vi "ImageGrabStatus.vi"(8 "error in (no error)":errorcluster, 11 "Image in":refnum<class "Image.lvclass">) -> (0 "error out":errorcluster, 2 "Stop?":bool, 3 "Image out":refnum<class "Image.lvclass">)   [LabVIEW 2012, in "Image.lvclass"]
uses:
  classes/Image.lvclass
  classes/Image.lvclass/Image.ctl
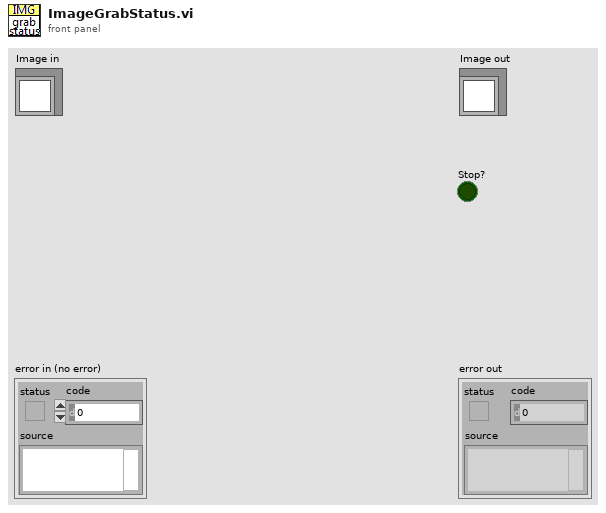
[diagram p1: front panel]
types:
  T1 = typedef "ScanMode.ctl" = enum16{"None", "Continuous", "Point Scan (CH3 cursor)", "Point Scan Move (CH3 cursor)", "Grab", "Grab Move Stage", "Grab Move Z-stage", "Cont. Move Z-stage", "Spec Move Stage", "Spec Move Cont", "Surf Calib"}
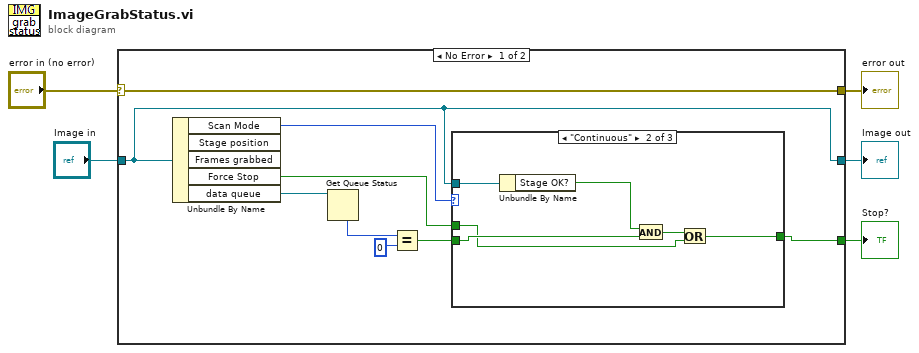
[diagram p0: block diagram]
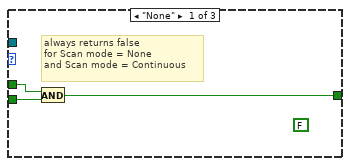
[diagram p2: hidden frame]
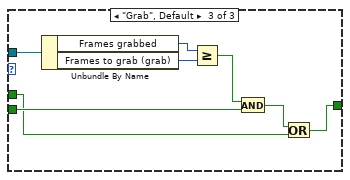
[diagram p3: hidden frame]
diagram:
  n1 = case shown="No Error" "error in (no error)" {
    selector: "error in (no error)" -> [w14 w33]
    tunnel: [w14 w33] -> w4
    tunnel: [w13 w32] -> w2
    tunnel: "Image in" -> [w13 w32]
    tunnel: [w6 _] -> w1
    frame No Error {
      n2 = Unbundle By Name(w13) -> ("Scan Mode"=w12:T1, "Force Stop"=w11:bool, "data queue"=w10:refnum<queue>)  [unwired: 2 out]
      n3 = Get Queue Status(queue=w10) -> (# elements in queue=w9:i32)  [unwired: 2 in, 7 out]
      n4 = Equal?(x=w9, y=0) -> (x = y?=w7:bool)
      n5 = case shown="\"Continuous\"" w12 {
        tunnel: [w15 w18 w24] -> w6
        tunnel: w13 -> [_ w23 w29]
        tunnel: w11 -> [w17 w19 w25]
        tunnel: w7 -> [w16 w21 w27]
        frame "None" {
          (unwired) FALSE
          # "always returns false\nfor Scan mode = None\nand Scan mode = Continuous"
          n6 = And(x=w17, y=w16) -> (x .and. y?=w15:bool)
        }
        frame "Continuous" {
          n7 = Unbundle By Name(w23) -> ("Stage OK?"=w22:bool)
          n8 = And(x=w22, y=w21) -> (x .and. y?=w20:bool)
          n9 = Or(x=w20, y=w19) -> (x .or. y?=w18:bool)
        }
        frame "Grab", Default {
          n10 = Unbundle By Name(w29) -> ("Frames grabbed"=w31:i32, "Frames to grab (grab)"=w30:i32)
          n11 = Greater Or Equal?(x=w31, y=w30) -> (x >= y?=w28:bool)
          n12 = And(x=w28, y=w27) -> (x .and. y?=w26:bool)
          n13 = Or(x=w26, y=w25) -> (x .or. y?=w24:bool)
        }
      }
    }
    frame Error {
    }
  }
  "error out" <- w4
  "Image out" <- w2
  "Stop?" <- w1
